vi "DMMsTest_2loops.vi"() -> ()   [LabVIEW 2017]
uses:
  DMMsData.lvclass
panel:
  out "error out 2":errorcluster
  in  "stop":bool
  out "current time":timestamp
  in  "Initialize":bool
  out "LastData":dbl[](array[numeric])
  out "DeviceActive?":bool[](array[boolean])
  out "XY Graph":T1(graph)
  in  "DMMsConfig":T2(array[cluster])
  out "DMMsLabels":string[](array[string])
  out "error out":errorcluster
  out "cycle #":i32
  out "RUN indicator":string
  in  "RUN label":string
  in  "base path":path
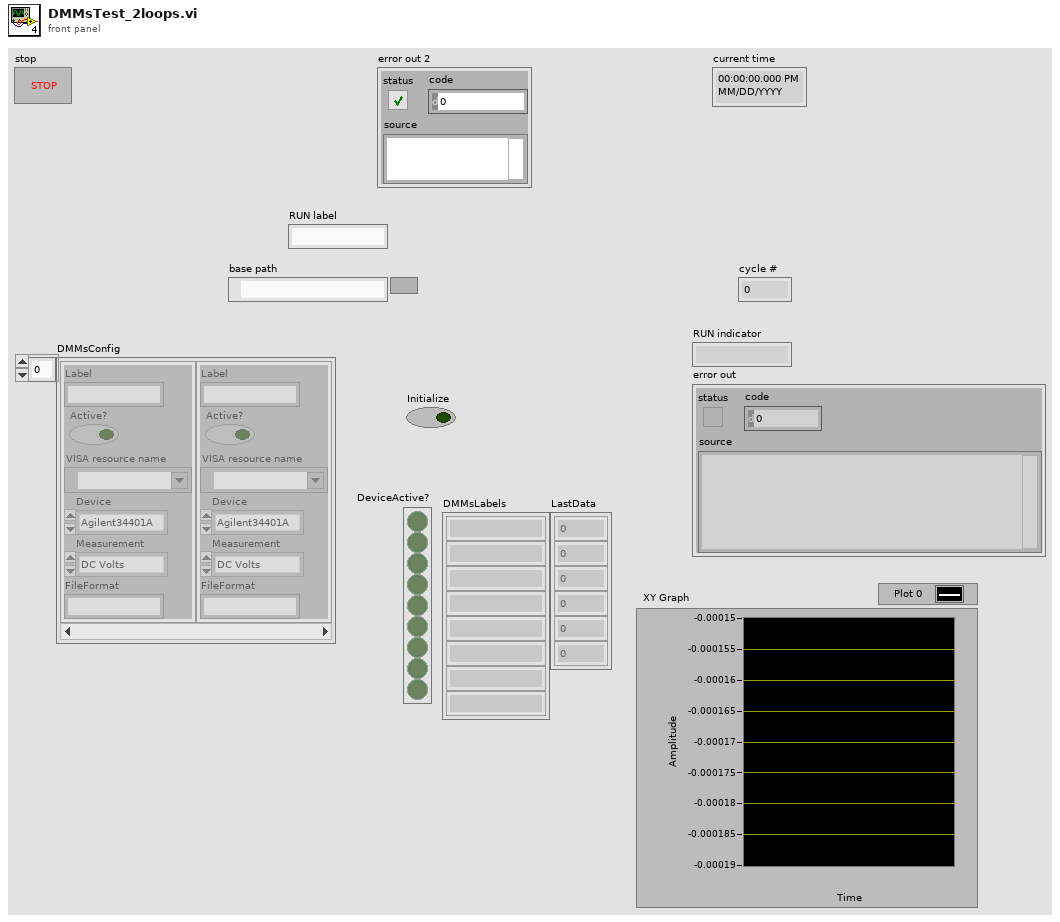
[diagram p1: front panel]
types:
  T1 = cluster{"TimeArray":timestamp[], "DataArray":dbl[]}[]
  T2 = cluster{"Label":string, "Active?":bool, "VISA resource name":refnum<visa-resource-name>, "Device":enum16{"Agilent34401A", "ADCMT7351", "HP3478A"}, "Measurement":enum16{"DC Volts", "DC Currents", "2-Wire Resistance", "4-Wire Resistance"}, "FileFormat":string}[]
  T3 = cluster{"TimeArray":timestamp[], "DataArray":dbl[]}
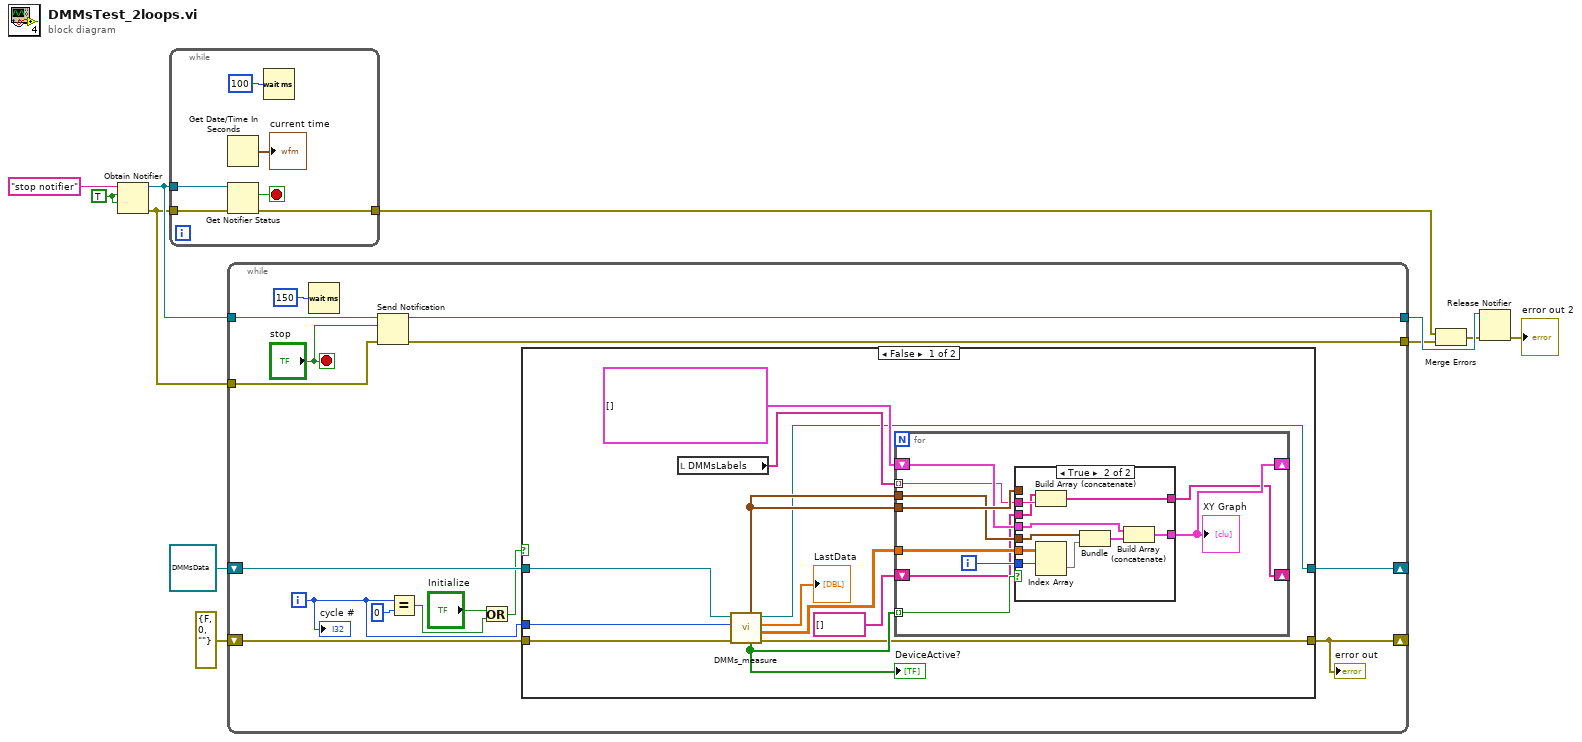
[diagram p0: block diagram]
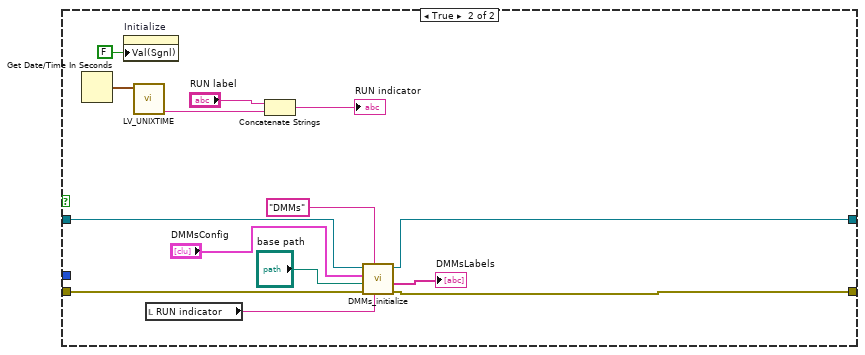
[diagram p3: hidden frame]
diagram:
  w7 = TRUE ("create if not found? (T)")
  n1 = Obtain Notifier(name (unnamed)="stop notifier", notification data type=w7, create if not found? (T)=w7) -> (notifier out=w9:refnum<notifier>, error out=w3:errorcluster)  [unwired: 1 in, 1 out]
  n2 = while {
    tunnel: w9 -> [w15]
    tunnel: [w13] -> w4
    tunnel: w3 -> [w12]
    stop <- w14 stop-if-true
    n3 = Get Date/Time In Seconds() -> (seconds since 1Jan1904=→"current time":timestamp)
    n4 = Get Notifier Status(notifier=w15, error in (no error)=w12) -> (current notification=w14:bool, error out=w13:errorcluster)  [unwired: 3 out]
    n5 = Wait (ms)(milliseconds to wait=u32 100) -> ()  [unwired: 1 out]
  }
  n6 = while {
    shift-right: [w26] -> _
    shift-left: refnum<class "DMMsData.lvclass"> refnum ("DMMsData in") -> [w29]
    shift-right: [w28] -> _
    shift-left: errorcluster {"status"=FALSE, "code"=0, "source"=""} ("error in (no error)") -> [w27]
    tunnel: w9 -> [w22]
    tunnel: [w21] -> w8
    tunnel: w3 -> [w20]
    tunnel: [w19] -> w5
    i -> [w30]
    stop <- "stop" stop-if-true
    n7 = Wait (ms)(milliseconds to wait=u32 150) -> ()  [unwired: 1 out]
    n8 = Send Notification(notification="stop", notifier=w22, error in (no error)=w20) -> (notifier out=w21:refnum<notifier>, error out=w19:errorcluster)
    n9 = Equal?(x=w30, y=0) -> (x = y?=w25:bool)
    n10 = Or(x="Initialize", y=w25) -> (x .or. y?=w24:bool)
    n11 = case shown="False" w24 {
      tunnel: w30 -> [w37 _]
      tunnel: w29 -> [w36 w70]
      tunnel: [w35 w71] -> w28
      tunnel: w27 -> [w33 w69]
      tunnel: [w34 w68] -> w26
      frame False {
        n12 = local read "DMMsLabels"() -> (w40:string[])
        n13 = call-dynamic "DMMs_measure.vi"("error in (no error)"=w33, "MeasurementIndex"=w37, "DMMsData in"=w36) -> ("error out"=w35:errorcluster, "DataArray"=w44:dbl[][], "LastData"=→"LastData":dbl[], "DMMsData out"=w34:refnum<class "DMMsData.lvclass">, "DeviceActive?"=w41:bool[], "TimeArray"=w43:timestamp[])  [unwired: 3 in]
        "DeviceActive?" <- w41
        n14 = for {
          tunnel: w43 -> [w54]
          shift-right: [w49] -> _
          shift-left: T1 [] -> [w53]
          tunnel: w44 -> [w52]
          tunnel: w43 -> [w51]
          tunnel: w41 -> [w48] mode=indexing
          shift-right: [w47] -> _
          shift-left: string[] [] -> [w45]
          tunnel: w40 -> [w46] mode=indexing
          i -> [w50]
          n15 = case shown="True" w48 {
            tunnel: w54 -> [_ _]
            tunnel: [w56 w66] -> w49
            tunnel: w53 -> [w56 w60]
            tunnel: w52 -> [_ w65]
            tunnel: w51 -> [_ w64]
            tunnel: w50 -> [_ w62]
            tunnel: [w55 w59] -> w47
            tunnel: w46 -> [_ w58]
            tunnel: w45 -> [w55 w57]
            frame False {
            }
            frame True {
              n16 = Build Array (concatenate)(w57, w58) -> (w59:string[])
              n17 = Index Array(array=w65, index (row)=w62) -> (element=w63:dbl[])  [unwired: 1 in]
              n18 = Bundle("TimeArray"=w64, "DataArray"=w63) -> (w61:T3)  [unwired: 1 in]
              n19 = Build Array (concatenate)(w60, w61) -> (w66:T1)
            }
          }
          "XY Graph" <- w49
        }
      }
      frame True {
        n20 = Get Date/Time In Seconds() -> (seconds since 1Jan1904=w77:timestamp)
        n21 = property on="Initialize" class="Bool (strict)"("Val(Sgnl)"=FALSE ("Value (Signaling)")) -> ()  [unwired: 2 in, 2 out]
        n22 = call "LV_UNIXTIME.vi"("current time"=w77) -> ("date/time string"=w78:string)  [unwired: 9 in, 1 out]
        n23 = local read "RUN indicator"() -> (w73:string)
        n24 = Concatenate Strings("RUN label", w78) -> (→"RUN indicator":string)
        n25 = call-dynamic "DMMs_initialize.vi"("RunIdentifier"=w73, "InstName"="DMMs", "error in (no error)"=w69, "base path"="base path", "DMMsConfig"="DMMsConfig", "DMMsData in"=w70) -> ("error out"=w71:errorcluster, "DMMsLabels"=→"DMMsLabels":string[], "DMMsData out"=w68:refnum<class "DMMsData.lvclass">)  [unwired: 2 in, 1 out]
      }
    }
    "error out" <- w28
    "cycle #" <- w30
  }
  n26 = Merge Errors(w4, w5) -> (w2:errorcluster)
  n27 = Release Notifier(notifier=w8, error in (no error)=w2) -> (error out=→"error out 2":errorcluster)  [unwired: 1 in, 2 out]
